vi "UiControls_gm.vi"() -> ()   [LabVIEW 2011]
uses:
  Output - Cluster gas.ctl
  gas_values.ctl
  Input - Cluster gas.ctl
panel:
  in  "Tab Control":enum32{"controls", "tools"}(tab)
  out "measuring volume":dbl
  in  "measuring point":u32(ring) items=["0"=0, "Fabes 2 MR"=1, "Fabes 2 HR"=2, "Fabes 1 MR"=4, "Fabes 1 BL"=8, "Fabes 1 HR"=16, "B2G 1 HR"=32, "B2G 1 T-2"=64, "B2G 1 MR"=128, "B2G 2 T-2"=256, "B2G 2 MR"=512, "calibration"=1024]
  in  "measuring mode":u8(ring) items=["quality & quantity"=3, "quality"=1, "quantity"=2, "0"=0, "flushing"=9]
  in  "start":bool
  in  "meas timetable":bool caption="activate"
  in  "timetable":string[][](table) caption="Zeitplan"
  out "measuring mode":u8
  in  "stop":bool caption="stop crio"
  out "pc":timestamp
  out "crio":timestamp
  in  "load/save":enum16{"Load", "Save"}(ring)
  in  "enter":bool
  in  "config file":path caption="path"
  out "status":string
  # "measuring mode :\n0: nothing\n1: quality (~7l)\n2: quantity (max. 700l)\n3: quality and quantity\n9: flushing"
  # "timestamp"
  # "configurtaion file"
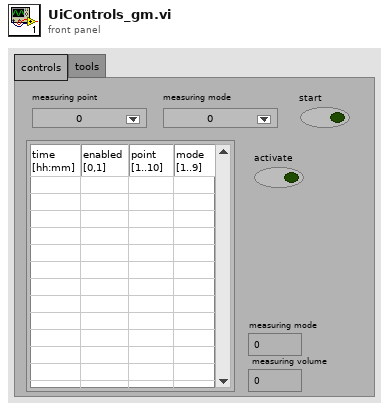
[diagram p1: front panel]
types:
  T1 = typedef "Output - Cluster gas.ctl" = cluster{"B2G2 MR V1.1 AUF":bool, "B2G2 MR V1.1 ZU":bool, "B2G2 MR V1 AUF":bool, "B2G2 MR V1 ZU":bool, "B2G1 T2 V1 AUF":bool, "B2G1 T2 V1 ZU":bool, "B2G1 T2 V1.1 AUF":bool, "B2G1 T2 V1.1 ZU":bool, "B2G2 T2 V1 AUF":bool, "B2G2 T2 V1 ZU":bool, "B2G2 T2 V1.1 ZU":bool, "B2G2 T2 V1.1 AUF":bool, "B2G1 MR V1 AUF":bool, "B2G1 MR V1 ZU":bool, "B2G1 MR V1.1 AUF":bool, "B2G1 MR V1.1 ZU":bool, "B2G1 HR V1 AUF":bool, "B2G1 HR V1 ZU":bool, "B2G1 HR V1.1 AUF":bool, "B2G1 HR V1.1 ZU":bool, "Fab1 HR V1 AUF":bool, "Fab1 HR V1 ZU":bool, "Fab1 HR V1.1 AUF":bool, "Fab1 HR V1.1 ZU":bool, "Fab1 MR V1 AUF":bool, "Fab1 MR V1 ZU":bool, "Fab1 MR V1.1 AUF":bool, "Fab1 MR V1.1 ZU":bool, "Fab1 BL V1 AUF":bool, "Fab1 BL V1 ZU":bool, "Fab1 BL V1.1 AUF":bool, "Fab1 BL V1.1 ZU":bool, "Fab2 HR V1 AUF":bool, "Fab2 HR V1 ZU":bool, "Fab2 HR V1.1 AUF":bool, "Fab2 HR V1.1 ZU":bool, "Fab2 MR V1 AUF":bool, "Fab2 MR V1 ZU":bool, "Fab2 MR V1.1 AUF":bool, "Fab2 MR V1.1 ZU":bool, "GA1 ch4 [%]":dbl, "GA1 co2 [%]":dbl, "GA1 h2 [%]":dbl, "GM P1 RUN":bool, "GM V-1 AUF":bool, "GM V-1 ZU":bool, "GM V-2 AUF":bool, "GM V-2 ZU":bool, "GM V-3 AUF":bool, "GM V-3 ZU":bool, "GM V-4 AUF":bool, "GM V-4 ZU":bool, "GM P2 RUN":bool, "GM GZ-1 [imp]":u32, "GM DS-2 [bar]":dbl, "GM DS-1 [bar]":dbl, "GM TS-1 [°C]":dbl, "GM TS-2[°C]":dbl, "gas_values":T2, "measuring mode":u8, "GM V-5":bool, "measuring volume":dbl, "automatic":bool}
  T2 = typedef "gas_values.ctl" = cluster{"start":timestamp, "GM DS-2 [bar]":dbl, "GA1 ch4 [%]":dbl, "GA1 co2 [%]":dbl, "GA1 h2 [%]":dbl, "GM DS-1 [bar]":dbl, "GM TS-1 [°C]":dbl, "GM TS-2 [°C]":dbl, "GM GZ-1 [l]":dbl, "measuring point":u8, "end":timestamp, "empty":bool, "GM GZ-1 [l] 2":dbl, "GM TS-1 [°C] 2":dbl, "GM DS-1 [bar] 2":dbl, "GM DS-2 [bar] 2":dbl, "empty 2":bool, "measuring mode":u8}
  T3 = enum8{"Enabled", "Disabled", "Disabled and Grayed Out"}
  T4 = typedef "Input - Cluster gas.ctl" = cluster{"GM P-1":bool, "GM P-2":bool, "measuring point":u32, "measuring mode":u8, "GM-V1,2":bool, "GM-V3,4":bool, "GM-V5":bool, "measuring volume":u32}
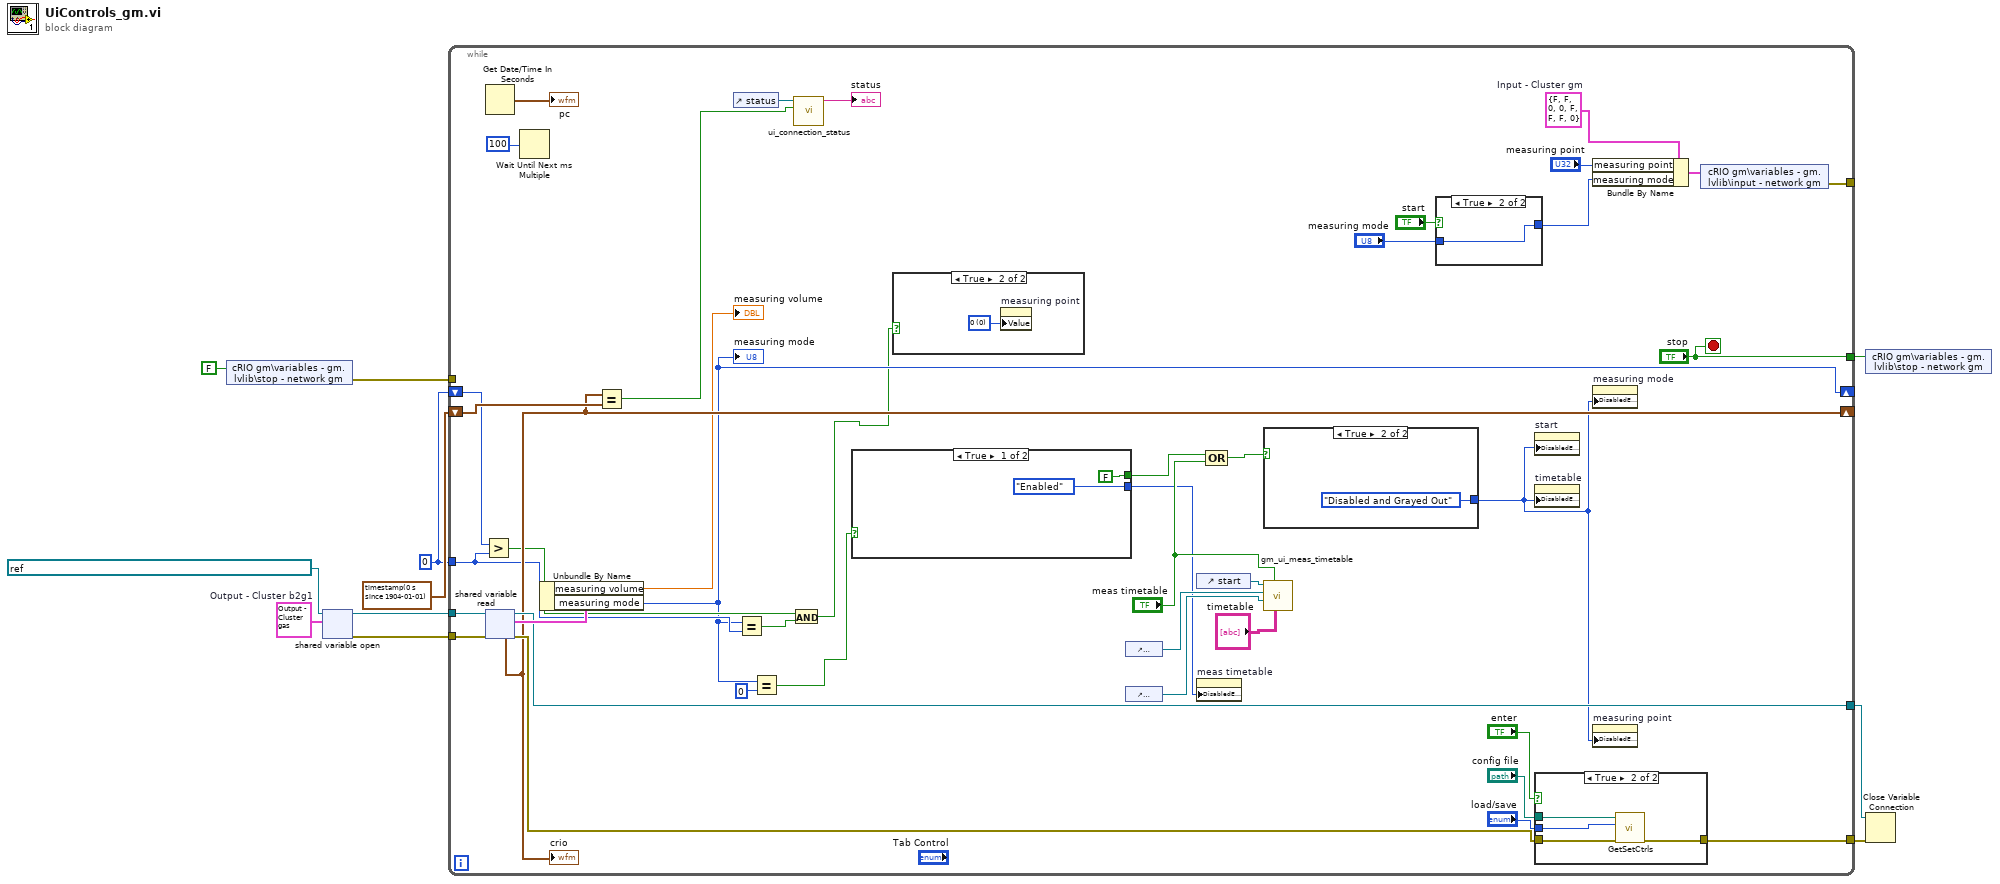
[diagram p0: block diagram]
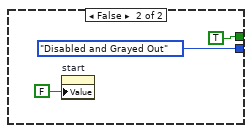
[diagram p3: hidden frame]
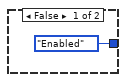
[diagram p4: hidden frame]
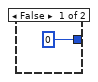
[diagram p5: hidden frame]
diagram:
  w1 = u8 0 ("y")
  w3 = T1 {"B2G2 MR V1.1 AUF"=FALSE, "B2G2 MR V1.1 ZU"=FALSE, "B2G2 MR V1 AUF"=FALSE, "B2G2 MR V1 ZU"=FALSE, "B2G1 T2 V1 AUF"=FALSE, "B2G1 T2 V1 ZU"=FALSE, "B2G1 T2 V1.1 AUF"=FALSE, "B2G1 T2 V1.1 ZU"=FALSE, "B2G2 T2 V1 AUF"=FALSE, "B2G2 T2 V1 ZU"=FALSE, "B2G2 T2 V1.1 ZU"=FALSE, "B2G2 T2 V1.1 AUF"=FALSE, "B2G1 MR V1 AUF"=FALSE, "B2G1 MR V1 ZU"=FALSE, "B2G1 MR V1.1 AUF"=FALSE, "B2G1 MR V1.1 ZU"=FALSE, "B2G1 HR V1 AUF"=FALSE, "B2G1 HR V1 ZU"=FALSE, "B2G1 HR V1.1 AUF"=FALSE, "B2G1 HR V1.1 ZU"=FALSE, "Fab1 HR V1 AUF"=FALSE, "Fab1 HR V1 ZU"=FALSE, "Fab1 HR V1.1 AUF"=FALSE, "Fab1 HR V1.1 ZU"=FALSE, "Fab1 MR V1 AUF"=FALSE, "Fab1 MR V1 ZU"=FALSE, "Fab1 MR V1.1 AUF"=FALSE, "Fab1 MR V1.1 ZU"=FALSE, "Fab1 BL V1 AUF"=FALSE, "Fab1 BL V1 ZU"=FALSE, "Fab1 BL V1.1 AUF"=FALSE, "Fab1 BL V1.1 ZU"=FALSE, "Fab2 HR V1 AUF"=FALSE, "Fab2 HR V1 ZU"=FALSE, "Fab2 HR V1.1 AUF"=FALSE, "Fab2 HR V1.1 ZU"=FALSE, "Fab2 MR V1 AUF"=FALSE, "Fab2 MR V1 ZU"=FALSE, "Fab2 MR V1.1 AUF"=FALSE, "Fab2 MR V1.1 ZU"=FALSE, "GA1 ch4 [%]"=0.0, "GA1 co2 [%]"=0.0, "GA1 h2 [%]"=0.0, "GM P1 RUN"=FALSE, "GM V-1 AUF"=FALSE, "GM V-1 ZU"=FALSE, "GM V-2 AUF"=FALSE, "GM V-2 ZU"=FALSE, "GM V-3 AUF"=FALSE, "GM V-3 ZU"=FALSE, "GM V-4 AUF"=FALSE, "GM V-4 ZU"=FALSE, "GM P2 RUN"=FALSE, "GM GZ-1 [imp]"=0, "GM DS-2 [bar]"=0.0, "GM DS-1 [bar]"=0.0, "GM TS-1 [°C]"=0.0, "GM TS-2[°C]"=0.0, "gas_values"={"start"=timestamp(0 s since 1904-01-01), "GM DS-2 [bar]"=0.0, "GA1 ch4 [%]"=0.0, "GA1 co2 [%]"=0.0, "GA1 h2 [%]"=0.0, "GM DS-1 [bar]"=0.0, "GM TS-1 [°C]"=0.0, "GM TS-2 [°C]"=0.0, "GM GZ-1 [l]"=0.0, "measuring point"=0, "end"=timestamp(0 s since 1904-01-01), "empty"=FALSE, "GM GZ-1 [l] 2"=0.0, "GM TS-1 [°C] 2"=0.0, "GM DS-1 [bar] 2"=0.0, "GM DS-2 [bar] 2"=0.0, "empty 2"=FALSE, "measuring mode"=0}, "measuring mode"=0, "GM V-5"=FALSE, "measuring volume"=0.0, "automatic"=FALSE}  # Output - Cluster b2g1
  n1 = shared-variable "cRIO gm\\variables - gm.lvlib\\stop - network gm"(FALSE ("stop - network")) -> (error out=w10:errorcluster)  [unwired: 1 in]
  n2 = shared-variable-open(refnum<k21> "ni.var.psp://10.27.40.21/variables - gm/data - network - gm" ("shared variable refnum in"), w3) -> (w7:refnum<k21>, w5:errorcluster)  [unwired: 2 in]
  n3 = while {
    tunnel: ["stop"] -> w11
    tunnel: w10 -> [_]
    tunnel: [w51] -> _
    tunnel: w7 -> [w48]
    tunnel: [w46] -> w6
    tunnel: w5 -> [w45]
    tunnel: [w41] -> w4
    shift-right: [w31] -> _
    shift-left: timestamp(0 s since 1904-01-01) -> [w32]
    shift-right: [w15] -> _
    shift-left: w1 -> [w20]
    tunnel: w1 -> [w17]
    stop <- "stop" stop-if-true
    w53 = T4 {"GM P-1"=FALSE, "GM P-2"=FALSE, "measuring point"=0, "measuring mode"=0, "GM-V1,2"=FALSE, "GM-V3,4"=FALSE, "GM-V5"=FALSE, "measuring volume"=0}  # Input - Cluster gm
    n4 = Greater?(x=w20, y=w17) -> (0:w19:bool)
    n5 = Get Date/Time In Seconds() -> (seconds since 1Jan1904=→"pc":timestamp)
    n6 = shared-variable-read(w48, w45) -> (w46:refnum<k21>, w42:errorcluster, w47:T1, w31:timestamp)
    "crio" <- w31
    n7 = Wait Until Next ms Multiple(millisecond multiple=u32 100) -> ()  [unwired: 1 out]
    n8 = Unbundle By Name(w47) -> ("measuring volume"=→"measuring volume":dbl, "measuring mode"=w15:u8)
    "measuring mode" <- w15
    n9 = Equal?(x=w31, y=w32) -> (x = y?=w35:bool)
    n10 = control-ref of="status"() -> (w34:refnum<vi>)
    n11 = Equal?(x=w15, y=w17) -> (x = y?=w18:bool)
    n12 = Equal?(x=w15, y=u8 0) -> (x = y?=w13:bool)
    n13 = And(x=w19, y=w18) -> (x .and. y?=w12:bool)
    n14 = call "ui_connection_status.vi"("Boolean"=w35, "String in"=w34) -> ("status"=→"status":string)  [unwired: 9 in]
    n15 = case shown="True" w13 {
      tunnel: [FALSE TRUE] -> w24
      tunnel: [T3."Enabled" ("Disabled") T3."Disabled and Grayed Out" ("Disabled")] -> w22
      frame True {
      }
      frame False {
        n16 = property on="start" class="Bool (strict)"("Value"=FALSE ("start")) -> ()  [unwired: 2 in, 2 out]
      }
    }
    n17 = case shown="True" w12 {
      frame False {
      }
      frame True {
        w54 = u32 0 items=["0"=0, "Fabes 2 MR"=1, "Fabes 2 HR"=2, "Fabes 1 MR"=4, "Fabes 1 BL"=8, "Fabes 1 HR"=16, "B2G 1 HR"=32, "B2G 1 T-2"=64, "B2G 1 MR"=128, "B2G 2 T-2"=256, "B2G 2 MR"=512] ("measuring point")
        n18 = property on="measuring point" class="Ring (strict)"("Value"=w54) -> ()  [unwired: 2 in, 2 out]
      }
    }
    n19 = control-ref of="measuring point"() -> (w27:refnum<vi>)
    n20 = control-ref of="measuring mode"() -> (w28:refnum<vi>)
    n21 = control-ref of="start"() -> (w29:refnum<vi>)
    n22 = property on="meas timetable" class="Bool (strict)"("DisabledEnum"=w22) -> ()  [unwired: 2 in, 2 out]
    n23 = Compound Arithmetic op=OR(w24, "meas timetable") -> (w25:bool)
    n24 = case shown="True" w25 {
      tunnel: [T3."Enabled" ("Disabled") T3."Disabled and Grayed Out" ("Disabled")] -> w23
      frame False {
      }
      frame True {
      }
    }
    n25 = call "gm_ui_meas_timetable.vi"("timetable"="timetable", "meas timetable"="meas timetable", "measuring mode"=w28, "measuring point"=w27, "Boolean in"=w29) -> ()  [unwired: 7 in]
    n26 = case shown="True" "start" {
      tunnel: [u8 0 ("measuring point") w63] -> w37
      tunnel: "measuring mode" -> [_ w63]
      frame False {
      }
      frame True {
      }
    }
    n27 = property on="start" class="Bool (strict)"("DisabledEnum"=w23) -> ()  [unwired: 2 in, 2 out]
    n28 = property on="timetable" class="Tbl (strict)"("DisabledEnum"=w23) -> ()  [unwired: 2 in, 2 out]
    n29 = case shown="True" "enter" {
      tunnel: w42 -> [w64 w68]
      tunnel: [w64 w67] -> w41
      tunnel: "load/save" -> [_ w66]
      tunnel: "config file" -> [_ w65]
      frame False {
      }
      frame True {
        n30 = call "GetSetCtrls.vi"("error in (no error)"=w68, "Function (Load)"=w66, "Ini file (empty)"=w65) -> ("error out"=w67:errorcluster)  [unwired: 8 in]
      }
    }
    n31 = Bundle By Name(cluster=w53, "measuring point"="measuring point", "measuring mode"=w37) -> (w52:T4)
    n32 = property on="measuring mode" class="Ring (strict)"("DisabledEnum"=w23) -> ()  [unwired: 2 in, 2 out]
    n33 = property on="measuring point" class="Ring (strict)"("DisabledEnum"=w23) -> ()  [unwired: 2 in, 2 out]
    n34 = shared-variable "cRIO gm\\variables - gm.lvlib\\input - network gm"(w52) -> (error out=w51:errorcluster)  [unwired: 1 in]
  }
  n35 = shared-variable "cRIO gm\\variables - gm.lvlib\\stop - network gm"(w11) -> ()  [unwired: 1 in, 1 out]
  n36 = Close Variable Connection(8:w4, 11:w6) -> ()  [unwired: 1 out]
